vi "FetchComic.vi"(8 "error in (no error)":errorcluster, 9 "Save to disk? (T)":bool=TRUE, 10 "ComicRootPath":path=path "C:/data/comics/comics", 11 "ComicURL":string) -> (0 "error out":errorcluster, 3 "Comic":T1 {"Cover Price" format="$%.2g"})   [LabVIEW 2022 SP3]
uses:
  TypeDefs/Comic.ctl
  TypeDefs/Character.ctl
  TypeDefs/Creator.ctl
  TypeDefs/Variant.ctl
  TypeDefs/LoCG_RootURL.ctl
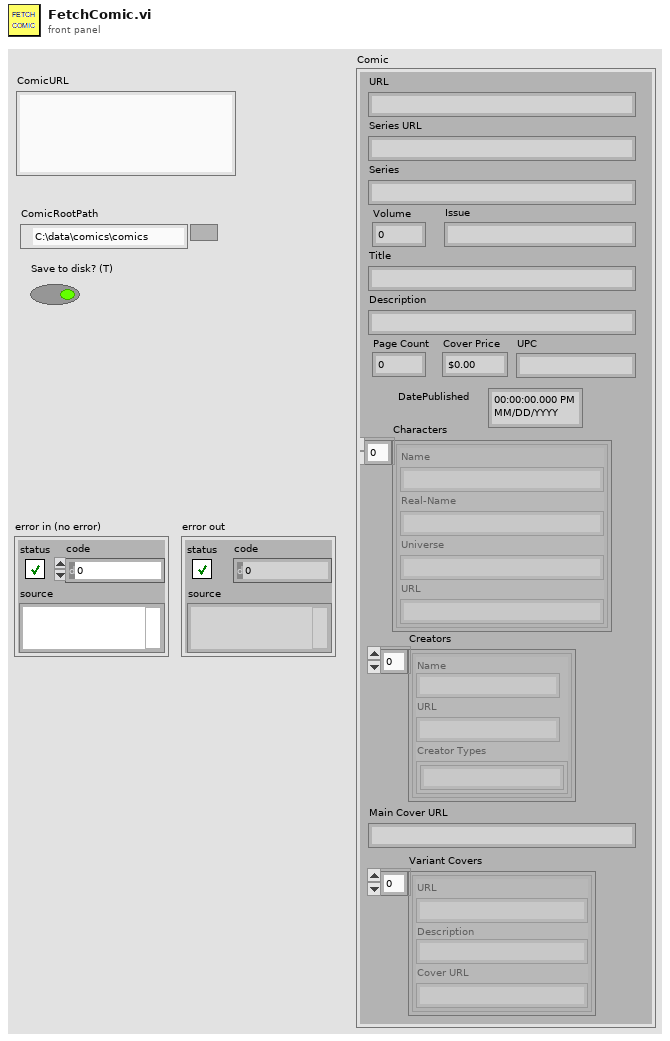
[diagram p1: front panel]
types:
  T1 = typedef "Comic.ctl" = cluster{"URL":string, "Series URL":string, "Series":string, "Volume":i32, "Issue":string, "Title":string, "Description":string, "Page Count":i32, "Cover Price":dbl, "UPC":string, "Characters":T2[], "Creators":T3[], "Main Cover URL":string, "Variant Covers":T4[], "DatePublished":timestamp}
  T2 = typedef "Character.ctl" = cluster{"Name":string, "Real-Name":string, "Universe":string, "URL":string}
  T3 = typedef "Creator.ctl" = cluster{"Name":string, "URL":string, "Creator Types":string[]}
  T4 = typedef "Variant.ctl" = cluster{"URL":string, "Description":string, "Cover URL":string}
  T5 = typedef "LoCG_RootURL.ctl" = string
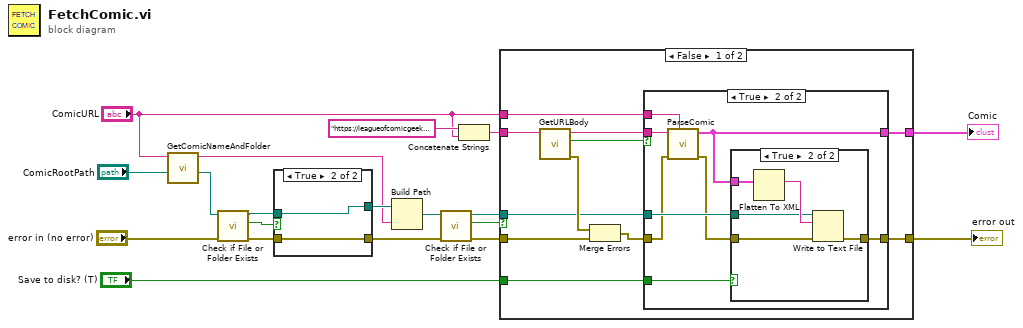
[diagram p0: block diagram]
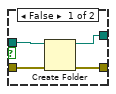
[diagram p2: hidden frame]
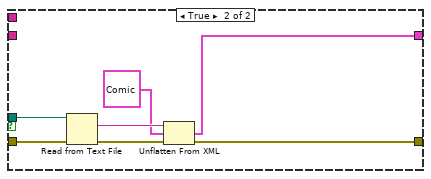
[diagram p5: hidden frame]
diagram:
  n1 = call "GetComicNameAndFolder.vi"("Local Path"="ComicRootPath", "URL"="ComicURL") -> ("OwningFolder"=w9:path, "FileName"=w8:string)  [unwired: 8 in]
  n2 = call <vilib>:"Check if File or Folder Exists.vi"("error in (no error)"="error in (no error)", "path"=w9) -> ("error out"=w13:errorcluster, "file or folder exists?"=w15:bool, "dup path"=w11:path)  [unwired: 7 in]
  n3 = case shown="True" w15 {
    tunnel: [w23 w25] -> w14
    tunnel: w13 -> [w22 w25]
    tunnel: [w20 w24] -> w12
    tunnel: w11 -> [w21 w24]
    frame False {
      n4 = Create Folder(path (use dialog)=w21, error in=w22) -> (created path=w20:path, error out=w23:errorcluster)  [unwired: 1 in, 1 out]
    }
    frame True {
    }
  }
  n5 = Build Path(base path=w12, name or relative path=w8) -> (appended path=w17:path)
  n6 = call <vilib>:"Check if File or Folder Exists.vi"("error in (no error)"=w14, "path"=w17) -> ("error out"=w19:errorcluster, "file or folder exists?"=w18:bool, "dup path"=w1:path)  [unwired: 7 in]
  n7 = Concatenate Strings(T5 "https://leagueofcomicgeeks.com/" ("LoCG Root Path"), "ComicURL") -> (w4:string)
  n8 = case shown="False" w18 {
    tunnel: w4 -> [w36 _]
    tunnel: w19 -> [w30 w58]
    tunnel: w1 -> [w27 w56]
    tunnel: [w33 w53] -> w7
    tunnel: [w29 w52] -> w6
    tunnel: "Save to disk? (T)" -> [w32 _]
    tunnel: "ComicURL" -> [w26 _]
    frame False {
      n9 = call "GetURLBody.vi"("URL"=w36) -> ("error out"=w31:errorcluster, "Success?"=w35:bool, "body"=w34:string)  [unwired: 7 in, 1 out]
      n10 = Merge Errors(w31, w30) -> (w28:errorcluster)
      n11 = case shown="True" w35 {
        tunnel: w34 -> [_ w45]
        tunnel: [_ w43] -> w33
        tunnel: w32 -> [_ w44]
        tunnel: [w37 w42] -> w29
        tunnel: w28 -> [w37 w39]
        tunnel: w27 -> [_ w41]
        tunnel: w26 -> [_ w40]
        frame False {
        }
        frame True {
          n12 = call "ParseComic.vi"("URL"=w40, "error in (no error)"=w39, "Issue"=w45) -> ("error out"=w38:errorcluster, "comic"=w43:T1)  [unwired: 7 in]
          n13 = case shown="True" w44 {
            tunnel: w43 -> [_ w51]
            tunnel: w38 -> [w46 w50]
            tunnel: [w46 w49] -> w42
            tunnel: w41 -> [_ w47]
            frame False {
            }
            frame True {
              n14 = Flatten To XML(6:w51) -> (2:w48:string)
              n15 = Write to Text File(file (use dialog)=w47, text=w48, error in=w50) -> (error out=w49:errorcluster)  [unwired: 1 in, 2 out]
            }
          }
        }
      }
    }
    frame True {
      n16 = Read from Text File(file (use dialog)=w56, error in=w58) -> (text=w57:string, error out=w54:errorcluster)  [unwired: 2 in, 2 out]
      n17 = Unflatten From XML(xml string=w57, type=T1 {"URL"="", "Series URL"="X-Factor", "Series"="", "Volume"=0, "Issue"="37", "Title"="", "Description"="https://s3.amazonaws.com/comicgeeks/comics/covers/large-5038184.jpg", "Page Count"=0, "Cover Price"=0.0, "UPC"="", "Characters"=[{"Name"="Beast", "Real-Name"="Henry McCoy", "Universe"="Earth-616", "URL"="/character/1568/beast"}, {"Name"="Cyclops", "Real-Name"="Scott Summers", "Universe"="Earth-616", "URL"="/character/279/cyclops"}, {"Name"="Dark Angel", "Real-Name"="Warren Worthington III", "Universe"="Earth-616", "URL"="/character/2252/dark-angel"}, {"Name"="Goblin Queen", "Real-Name"="Madelyne Pryor", "Universe"="Earth-616", "URL"="/character/2291/goblin-queen"}, {"Name"="Iceman", "Real-Name"="Bobby Drake", "Universe"="Earth-616", "URL"="/character/1570/iceman"}, {"Name"="Marvel Girl", "Real-Name"="Jean Grey", "Universe"="Earth-616", "URL"="/character/106/marvel-girl"}, {"Name"="N&#39;astirh", "Real-Name"="", "Universe"="Earth-616", "URL"="/character/7497/nastirh"}, {"Name"="Nathan Summers", "Real-Name"="", "Universe"="Earth-616", "URL"="/character/129/nathan-summers"}, {"Name"="Wolverine", "Real-Name"="James Howlett", "Universe"="Earth-616", "URL"="/character/48/wolverine"}], "Creators"=[], "Main Cover URL"="", "Variant Covers"=[], "DatePublished"=timestamp(0 s since 1904-01-01)} ("Comic"), error in (no error)=w54) -> (value=w53:T1, error out=w52:errorcluster)
    }
  }
  "error out" <- w6
  "Comic" <- w7
